vi "Release RC Override.vi"(8 "error in (no error)":errorcluster, 11 "Aircraft ID":u8) -> (0 "error out":errorcluster)   [LabVIEW 2014]
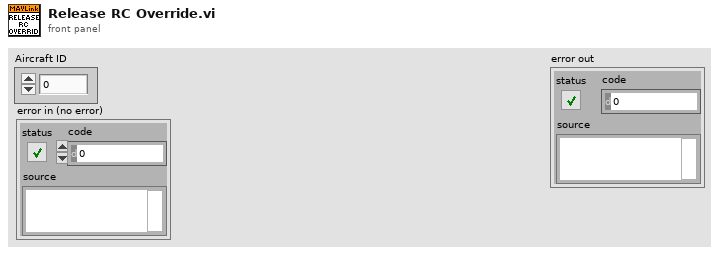
[diagram p1: front panel]
types:
  T1 = cluster{"chan1_raw":u16, "chan2_raw":u16, "chan3_raw":u16, "chan4_raw":u16, "chan5_raw":u16, "chan6_raw":u16, "chan7_raw":u16, "chan8_raw":u16, "target_system":u8, "target_component":u8}
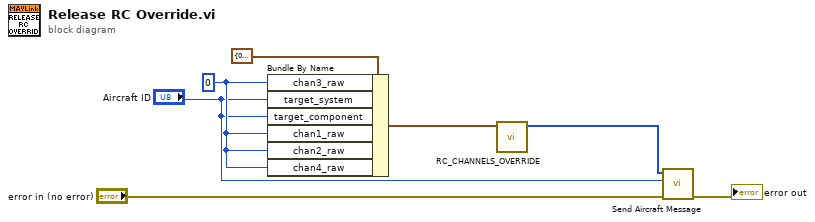
[diagram p0: block diagram]
diagram:
  w5 = u16 0 ("chan3_raw")
  n1 = Bundle By Name(cluster=T1 {"chan1_raw"=0, "chan2_raw"=0, "chan3_raw"=0, "chan4_raw"=0, "chan5_raw"=0, "chan6_raw"=0, "chan7_raw"=0, "chan8_raw"=0, "target_system"=0, "target_component"=0} ("Payload"), "chan3_raw"=w5, "target_system"="Aircraft ID", "target_component"="Aircraft ID", "chan1_raw"=w5, "chan2_raw"=w5, "chan4_raw"=w5) -> (w7:T1)
  n2 = call "RC_CHANNELS_OVERRIDE.vi"("Payload"=w7) -> ("MAVLink Message"=w4:u8[])  [unwired: 10 in]
  n3 = call "Send Aircraft Message.vi"("error in (no error)"="error in (no error)", "Aircraft ID"="Aircraft ID", "MAVLink Message"=w4) -> ("error out"=→"error out":errorcluster)  [unwired: 8 in]
